vi "generate_population2.vi"(11 "lambda":dbl format="%#_13g") -> (3 "Array":T1[](array[typedef]))   [LabVIEW 2014]
uses:
  Client.ctl
  LukiBrary.lvlib
  <vilib>/Analysis/NI_AALPro.lvlib
panel:
  out "derivative":dbl[](graph)
  out "Times":i32[](graph)
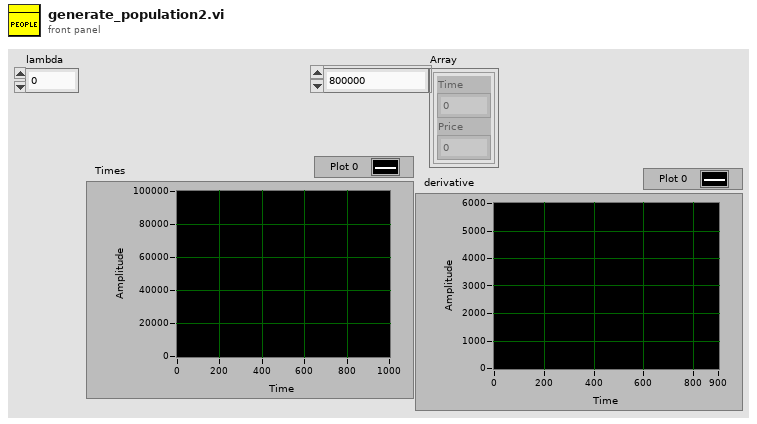
[diagram p1: front panel]
types:
  T1 = typedef "LukiBrary.lvlib/Client.ctl" = cluster{"Time":i32, "Price":i32}
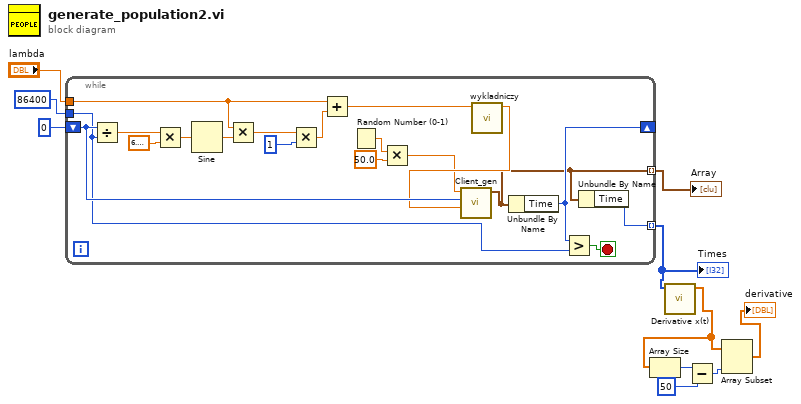
[diagram p0: block diagram]
diagram:
  n1 = while {
    shift-right: [w13] -> _
    shift-left: 0 -> [w18]
    tunnel: 86400 ("Czas") -> [w14]
    tunnel: "lambda" -> [w23]
    tunnel: [w12] -> w1 mode=indexing
    tunnel: [w11] -> w7 mode=indexing
    stop <- w15 stop-if-true
    n2 = Divide(x=w18, y=w14) -> (x/y=w27:dbl)
    n3 = Multiply(x=w27, y=6.283185307179586) -> (x*y=w25:dbl)
    n4 = Sine(x=w25) -> (sin(x)=w24:dbl)
    n5 = Multiply(x=w23, y=w24) -> (x*y=w21:dbl)
    n6 = Multiply(x=w21, y=1) -> (x*y=w22:dbl)
    n7 = Add(x=w23, y=w22) -> (x+y=w19:dbl)
    n8 = Random Number (0-1)() -> (number: 0 to 1=w29:dbl)
    n9 = Multiply(x=w29, y=50.0) -> (x*y=w16:dbl)
    n10 = call "wykladniczy.vi"("lambda"=w19) -> ("X~wykładniczy"=w17:dbl)  [unwired: 10 in]
    n11 = call "Client_gen.vi"("Różnica"=w17, "Time"=w18, "Price"=w16) -> ("Client"=w12:T1)  [unwired: 8 in]
    n12 = Unbundle By Name(w12) -> ("Time"=w13:i32)
    n13 = Greater?(x=w13, y=w14) -> (0:w15:bool)
    n14 = Unbundle By Name(w12) -> ("Time"=w11:i32)
  }
  "Array" <- w1
  "Times" <- w7
  n15 = call <vilib>:"Derivative x(t).vi"("X"=w7) -> ("dX/dt"=w3:dbl[])  [unwired: 9 in, 1 out]
  n16 = Array Size(array=w3) -> (size(s)=w6:i32)
  n17 = Subtract(x=w6, y=50) -> (x-y=w4:i32)
  n18 = Array Subset(array=w3, length=w4) -> (→"derivative":dbl[])  [unwired: 1 in]
